vi "Copy Scripting API to Installed Location.vi"(5 "Files Generated by Build":path[](array[path]), 6 "Top Level/Always Included VIs":path[](array[path]), 7 "Destination Path":path, 8 "error in (no error)":errorcluster, 9 "Target Name":string, 10 "Build Specification Name":string, 11 "Project Path":path) -> (0 "error out":errorcluster)   [LabVIEW 2017]
doc: "This VI is called after each run of a build specification. The VI will copy the generated LLB (Engine or System Explorer) into the VeriStand Custom Device folder (...\\Documents\\National Instruments\\NI VeriStand 2013...)."
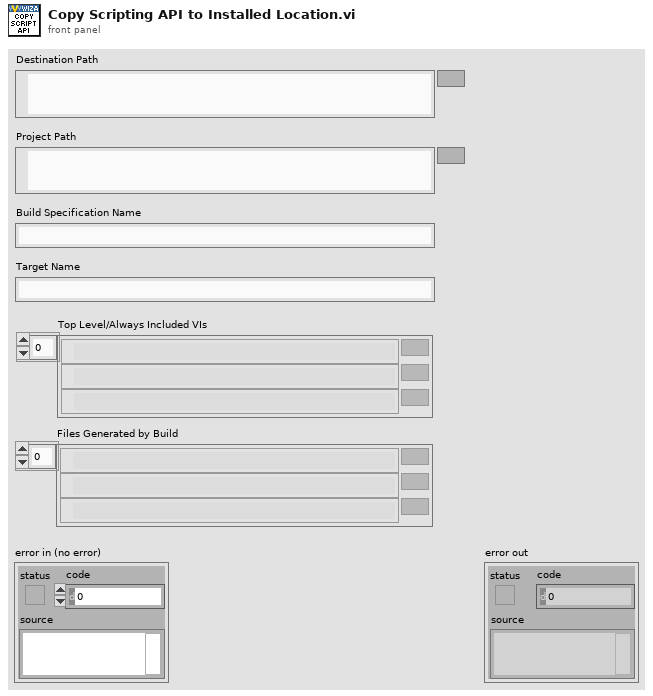
[diagram p1: front panel]
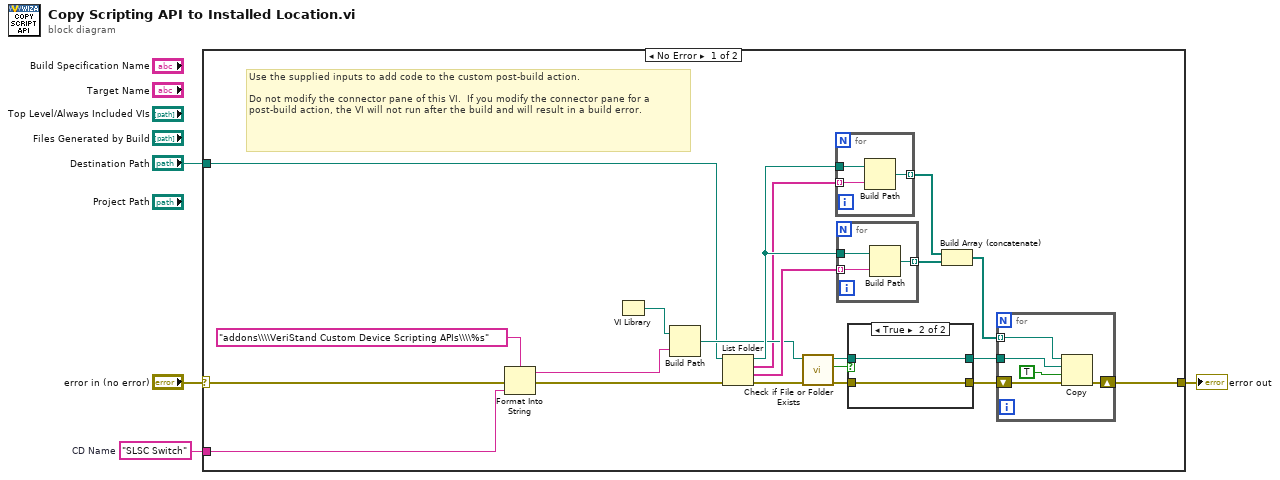
[diagram p0: block diagram]
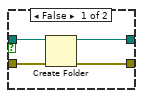
[diagram p2: hidden frame]
diagram:
  w3 = "SLSC Switch"  # CD Name
  n1 = case shown="No Error" "error in (no error)" {
    selector: "error in (no error)" -> [w13 w43]
    tunnel: [w5 w43] -> w2
    tunnel: w3 -> [w11 _]
    tunnel: "Destination Path" -> [w6 _]
    frame No Error {
      # "Use the supplied inputs to add code to the custom post-build action.\n\nDo not modify the connector pane of this VI.  If you modify the connector pane for a post-build action, the VI will not run after the build and will result in a build error."
      n2 = Format Into String(format string="addons\\\\VeriStand Custom Device Scripting APIs\\\\%s" ("name or relative path"), error in=w13, w11) -> (resulting string=w16:string, error out=w12:errorcluster)  [unwired: 1 in]
      n3 = VI Library() -> (path=w7:path)
      n4 = Build Path(base path=w7, name or relative path=w16) -> (appended path=w14:path)
      n5 = List Folder(path=w6, error in=w12) -> (path out=w19:path, filenames=w9:string[], folder names=w20:string[], error out=w17:errorcluster)  [unwired: 2 in]
      n6 = call <vilib>:"Check if File or Folder Exists.vi"("error in (no error)"=w17, "path"=w14) -> ("error out"=w21:errorcluster, "file or folder exists?"=w23:bool, "dup path"=w22:path)  [unwired: 7 in]
      n7 = for {
        tunnel: w9 -> [w41] mode=indexing
        tunnel: w19 -> [w42]
        tunnel: [w40] -> w25 mode=indexing
        n8 = Build Path(base path=w42, name or relative path=w41) -> (appended path=w40:path)
      }
      n9 = for {
        tunnel: w20 -> [w38] mode=indexing
        tunnel: w19 -> [w39]
        tunnel: [w37] -> w18 mode=indexing
        n10 = Build Path(base path=w39, name or relative path=w38) -> (appended path=w37:path)
      }
      n11 = case shown="True" w23 {
        tunnel: w22 -> [w29 w31]
        tunnel: w21 -> [w28 w30]
        tunnel: [w27 w31] -> w8
        tunnel: [w26 w30] -> w10
        frame False {
          n12 = Create Folder(path (use dialog)=w29, error in=w28) -> (created path=w27:path, error out=w26:errorcluster)  [unwired: 1 in, 1 out]
        }
        frame True {
        }
      }
      n13 = Build Array (concatenate)(w25, w18) -> (w24:path[])
      n14 = for {
        tunnel: w24 -> [w33] mode=indexing
        shift-right: [w34] -> w5
        shift-left: w10 -> [w35]
        tunnel: w8 -> [w32]
        n15 = Copy(8:w35, 9:TRUE ("overwrite (F)"), 10:w32, 11:w33) -> (0:w34:errorcluster)  [unwired: 1 in, 2 out]
      }
    }
    frame Error {
    }
  }
  "error out" <- w2
